vi "Get pos axis.vi"(8 "error in (no error)":errorcluster, 10 "Axis":i32=1 min=1 max=4, 11 "DLOwis in":refnum<class "DLOwis.lvclass">) -> (0 "error out":errorcluster, 2 "Pos":dbl, 3 "DLOwis out":refnum<class "DLOwis.lvclass">)   [LabVIEW 2018, in "DLOwis.lvclass"]
uses:
  DLOwis.lvclass
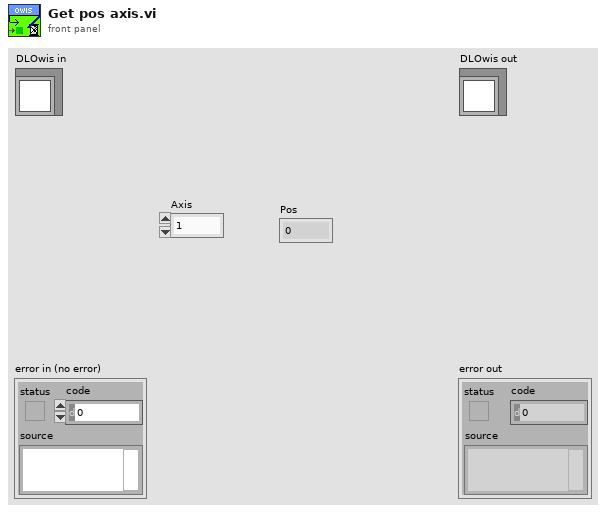
[diagram p1: front panel]
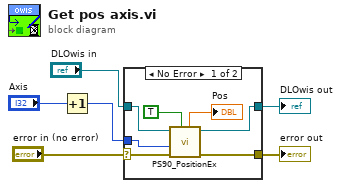
[diagram p0: block diagram]
diagram:
  n1 = Increment(x="Axis") -> (x+1=w1:i32)
  n2 = case shown="No Error" "error in (no error)" {
    selector: "error in (no error)" -> [w9 w15]
    tunnel: [w7 w15] -> w5
    tunnel: [w12 w14] -> w4
    tunnel: "DLOwis in" -> [w8 w14]
    tunnel: w1 -> [w11 _]
    frame No Error {
      n3 = call "PS90_PositionEx.vi"("read?"=TRUE, "error in (no error)"=w9, "Axis number"=w11, "DLOwis.lvclass"=w8) -> ("error out"=w7:errorcluster, "DLOwis.lvclass"=w12:refnum<class "DLOwis.lvclass">, "dValue-Out"=→"Pos":dbl)  [unwired: 4 in]
    }
    frame Error {
    }
  }
  "error out" <- w5
  "DLOwis out" <- w4
